vi "Get Arm Setpoint from Enum.vi"(8 "error in (no error)":errorcluster, 11 "Arm Mode":T1) -> (0 "error out":errorcluster, 3 "Angle":dbl, 5 "Enable Lock":bool)   [LabVIEW 2015]
uses:
  Arm Mode TypeDef.ctl
  <vilib>/Rock Robotics/Network Tables/NT Read Number.vi
  <vilib>/Rock Robotics/Network Tables/NT Read String.vi
  Global Variables.vi
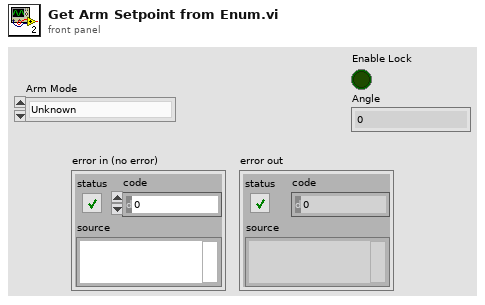
[diagram p1: front panel]
types:
  T1 = typedef "Arm Mode TypeDef.ctl" = enum16{"Unknown", "Disabled", "Locked", "Shoot Batter", "Shoot Close", "Cross Defense", "Human Player Load", "Low Bar / Goal", "Manual"}
  T2 = typedef "Arm Notifier TypeDef.ctl" = cluster{"Arm Mode":T1, "Manual Arm Angle":dbl}
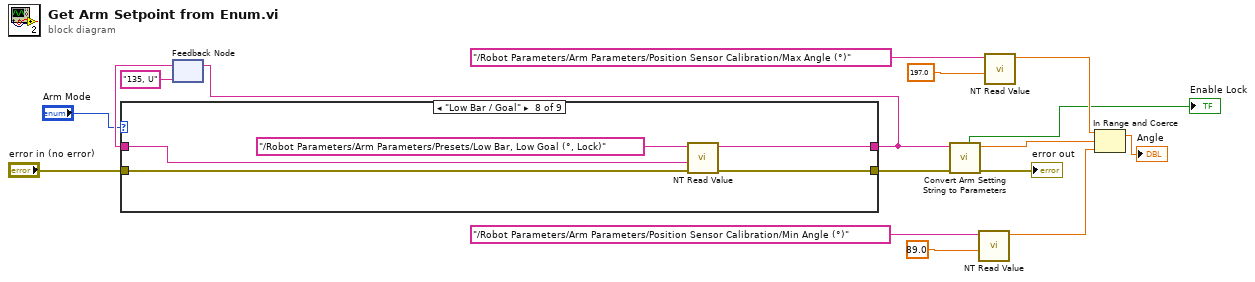
[diagram p0: block diagram]
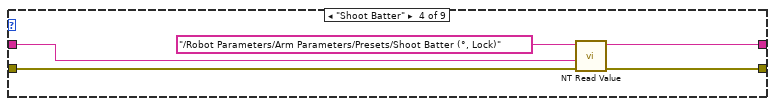
[diagram p5: hidden frame]
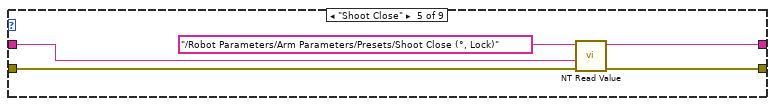
[diagram p6: hidden frame]
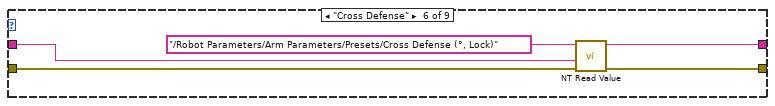
[diagram p7: hidden frame]
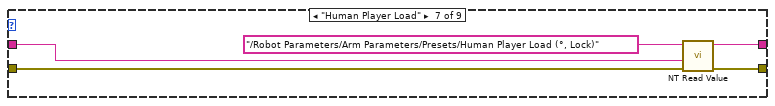
[diagram p8: hidden frame]
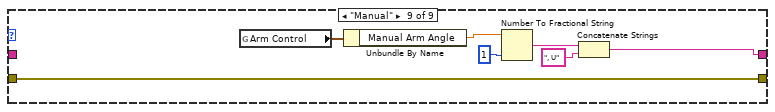
[diagram p9: hidden frame]
diagram:
  n1 = feedback #1("135, U") -> (w15:string)
  n2 = case shown="\"Low Bar / Goal\"" "Arm Mode" {
    tunnel: [w18 w20 w22 w25 w32 w37 w41 w46 w49] -> w14
    tunnel: w15 -> [w18 w20 w22 w26 w30 w35 w40 w45 _]
    tunnel: "error in (no error)" -> [w17 w19 w21 w24 w29 w34 w39 w44 w48]
    tunnel: [w17 w19 w21 w23 w28 w33 w38 w43 w48] -> w11
    frame "Unknown", Default {
    }
    frame "Disabled" {
    }
    frame "Locked" {
    }
    frame "Shoot Batter" {
      n3 = call-poly <vilib>:"NT Read Value.vi"("error in"=w24, "Default Value"=w26, "Name"="/Robot Parameters/Arm Parameters/Presets/Shoot Batter (°, Lock)") -> ("error out"=w23:errorcluster, "String"=w25:string)  [unwired: 7 in]
    }
    frame "Shoot Close" {
      n4 = call-poly <vilib>:"NT Read Value.vi"("error in"=w29, "Default Value"=w30, "Name"="/Robot Parameters/Arm Parameters/Presets/Shoot Close (°, Lock)") -> ("error out"=w28:errorcluster, "String"=w32:string)  [unwired: 7 in]
    }
    frame "Cross Defense" {
      n5 = call-poly <vilib>:"NT Read Value.vi"("error in"=w34, "Default Value"=w35, "Name"="/Robot Parameters/Arm Parameters/Presets/Cross Defense (°, Lock)") -> ("error out"=w33:errorcluster, "String"=w37:string)  [unwired: 7 in]
    }
    frame "Human Player Load" {
      n6 = call-poly <vilib>:"NT Read Value.vi"("error in"=w39, "Default Value"=w40, "Name"="/Robot Parameters/Arm Parameters/Presets/Human Player Load (°, Lock)") -> ("error out"=w38:errorcluster, "String"=w41:string)  [unwired: 7 in]
    }
    frame "Low Bar / Goal" {
      n7 = call-poly <vilib>:"NT Read Value.vi"("error in"=w44, "Default Value"=w45, "Name"="/Robot Parameters/Arm Parameters/Presets/Low Bar, Low Goal (°, Lock)") -> ("error out"=w43:errorcluster, "String"=w46:string)  [unwired: 7 in]
    }
    frame "Manual" {
      n8 = global read "Global Variables.vi" "Arm Control"() -> (w54:T2)
      n9 = Unbundle By Name(w54) -> ("Manual Arm Angle"=w53:dbl)
      n10 = Number To Fractional String(number=w53, precision (6)=i16 1) -> (F-format string=w51:string)  [unwired: 2 in]
      n11 = Concatenate Strings(w51, ", U" ("string")) -> (w49:string)
    }
  }
  n12 = feedback-in #1(w14) -> ()
  n13 = call "Convert Arm Setting String to Parameters.vi"("error in (no error)"=w11, "Arm Mode Setting"=w14) -> ("error out"=→"error out":errorcluster, "Angle"=w5:dbl, "Enable Lock"=→"Enable Lock":bool)  [unwired: 5 in]
  n14 = call-poly <vilib>:"NT Read Value.vi"("Default Value"=89.0, "Name"="/Robot Parameters/Arm Parameters/Position Sensor Calibration/Min Angle (°)") -> ("Numeric"=w2:dbl)  [unwired: 8 in, 1 out]
  n15 = call-poly <vilib>:"NT Read Value.vi"("Default Value"=197.0, "Name"="/Robot Parameters/Arm Parameters/Position Sensor Calibration/Max Angle (°)") -> ("Numeric"=w3:dbl)  [unwired: 8 in, 1 out]
  n16 = In Range and Coerce(upper limit=w3, x=w5, lower limit=w2) -> (coerced(x)=→"Angle":dbl)  [unwired: 1 out]
